vi "Test_BufferedLogBufferTimeout_EventsCaptured.vi"(8 "error in (no error)":errorcluster, 11 "TestCase in":refnum<class "TestBufferedLogSink.lvclass">) -> (0 "error out":errorcluster, 3 "TestCase out":refnum<class "TestBufferedLogSink.lvclass">)   [LabVIEW 2019, in "TestBufferedLogSink.lvclass"]
uses:
  TestBufferedLogSink.lvclass
  Source/Composed Log/LoggerReference/LoggerReference.lvclass/LoggerReference.ctl
  Source/LVQueue Sink/LVQueue Sink.lvclass/LVQueue Sink.ctl
  b83ac39a-525a-4956-83d8-1e446c51aff0.vi
  Source/Composed Log/LoggerReference/Return Aggregate Queues.vi
  Source/Composed Log/LoggerReference/Add Aggregate Log.vi
  b83ac39a-525a-4956-83d8-1e446c51aff0.vi/dcd4c0e4-37c7-45d5-9225-2a129c6cfbb9.vi
  Source/Composed Log/LoggerReference/Log.vi
  Source/Composed Log/LoggerReference/Get Valid Event Time.vi
  Source/Composed Log/LoggerReference/Send Add Sink.vi
  Source/Composed Log/LoggerReference/Remove Stale Logs.vi
  Source/LVQueue Sink/LVQueue Sink.lvclass
  C:/CS/Log/Source/Composed Log/Log Sink/Log Sink.lvclass
  Source/Buffered Log Sink/Buffered Log Sink.lvclass
  Source/Composed Log/Application Logger/Launch Worker Loop.vi
  Source/Composed Log/LoggerReference/Initialize Logger Instance.vi
  Source/Composed Log/LoggerReference/LoggerReference.lvclass
  Source/Composed Log/IErrorFormat/IErrorFormat.lvclass
  Source/Composed Log/Log Sink/Log Sink.lvclass
  <vilib>/addons/_JKI Toolkits/VI Tester/TestCase.llb/TestCase.lvclass
  C:/Program Files (x86)/National Instruments/LabVIEW 2019/vi.lib/addons/_JKI Toolkits/VI Tester/TestCase.llb/TestCase.lvclass
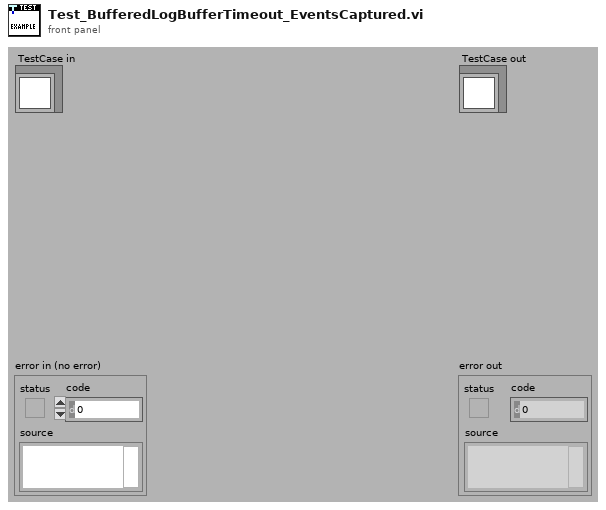
[diagram p1: front panel]
types:
  T1 = typedef "Composed Log.lvlib/Log Packet.ctl" = cluster{"Data To Log":string, "Source":string, "Event Level":T2, "Event Time":timestamp}
  T2 = typedef "Composed Log.lvlib/Log Level.ctl" = enum16{"Debug", "Info", "Warning", "Error", "Critical"}
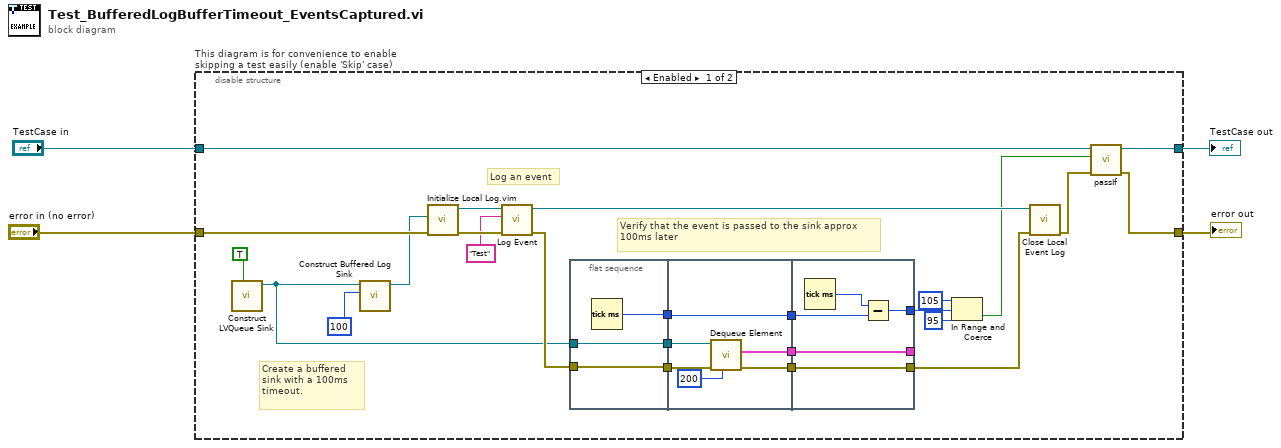
[diagram p0: block diagram]
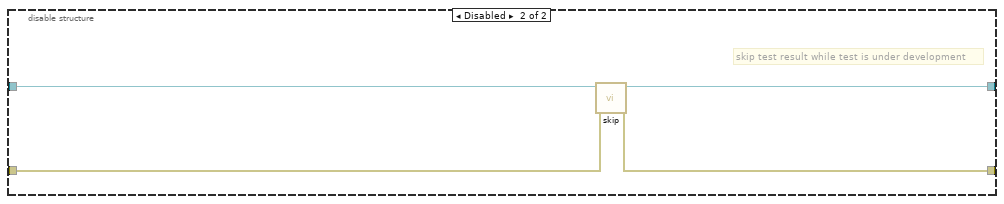
[diagram p2: hidden frame]
diagram:
  n1 = disable-structure "This diagram is for convenience to enable skipping a test easily (enable 'Skip' case)" shown="Enabled" {
    disable-tunnel: "TestCase in" -> [w11 w47]
    disable-tunnel: [w10 w45] -> w1
    disable-tunnel: [w9 w46] -> w3
    disable-tunnel: "error in (no error)" -> [w6 w44]
    frame Enabled {
      # "Verify that the event is passed to the sink approx 100ms later"
      # "Log an event"
      # "Create a buffered sink with a 100ms timeout."
      n2 = call "Construct LVQueue Sink.vi"("User Shutdown? (F)"=TRUE) -> ("LVQueue Sink out"=w22:refnum<class "LVQueue Sink.lvclass">)  [unwired: 9 in, 1 out]
      n3 = call "Construct Buffered Log Sink.vi"("Buffer Timeout ms (-1)"=100, "Sink to Buffer"=w22) -> ("Buffered Log Sink out"=w5:refnum<class "Buffered Log Sink.lvclass">)  [unwired: 9 in]
      n4 = call "Initialize Local Log.vim"("error in (no error)"=w6, "Startup Sink(s)"=w5) -> ("error out"=w29:errorcluster, "Log Instance Reference"=w28:refnum<class "LoggerReference.lvclass">)  [unwired: 7 in, 1 out]
      n5 = call "Log Event.vi"("error in (no error)"=w29, "SourceID"="Test", "Log Instance"=w28) -> ("error out"=w25:errorcluster, "Log Instance Out"=w27:refnum<class "LoggerReference.lvclass">)  [unwired: 7 in]
      n6 = flat-sequence {
        tunnel: w25 -> [w32]
        tunnel: [w32] -> w24
        tunnel: w22 -> [w31]
        tunnel: [w31] -> w21
        tunnel: [w30] -> w19
        tunnel: w24 -> [w37]
        tunnel: w21 -> [w38]
        tunnel: w19 -> [w33]
        tunnel: [w36] -> w18
        tunnel: [w35] -> w17
        tunnel: [w33] -> w16
        tunnel: [w42] -> _
        tunnel: [w43] -> w15
        tunnel: w18 -> [w43]
        tunnel: w17 -> [w42]
        tunnel: w16 -> [w40]
        tunnel: [w39] -> w14
        frame #0 {
          n7 = Tick Count (ms)() -> (millisecond timer value=w30:u32)
        }
        frame #1 {
          n8 = call "Dequeue Element.vi"("timeout in ms (-1)"=200, "error in (no error)"=w37, "LVQueue Sink in"=w38) -> ("error out"=w36:errorcluster, "Log Packet"=w35:T1)  [unwired: 5 in, 2 out]
        }
        frame #2 {
          n9 = Tick Count (ms)() -> (millisecond timer value=w41:u32)
          n10 = Subtract(x=w41, y=w40) -> (x-y=w39:u32)
        }
      }
      n11 = In Range and Coerce(upper limit=u32 105, x=w14, lower limit=u32 95) -> (In Range?=w7:bool)  [unwired: 1 out]
      n12 = call "Close Local Event Log.vi"("error in (no error)"=w15, "Log Instance"=w27) -> ("error out"=w8:errorcluster)  [unwired: 9 in]
      n13 = call-dynamic "passIf.vi"("error in (no error)"=w8, "pass"=w7, "TestCase in"=w11) -> ("error out"=w9:errorcluster, "TestCase out"=w10:refnum<class "TestBufferedLogSink.lvclass">)  [unwired: 7 in]
    }
    frame Disabled {
      # "skip test result while test is under development"
      n14 = call <vilib>:"skip.vi"("error in (no error)"=w44, "TestCase in"=w47) -> ("error out"=w46:errorcluster, "TestCase out"=w45:refnum<class "TestBufferedLogSink.lvclass">)  [unwired: 8 in]
    }
  }
  "error out" <- w3
  "TestCase out" <- w1
